vi "CalcFC.vi"(1 "CapUnits":u16(ring) items=["uF", "nF", "pF"], 2 "ResistorUnits":i32(ring) items=["ohm", "Kohm "], 3 "C":ext format="%#_6f", 4 "R":ext format="%#_6f") -> (0 "Fc":ext)   [LabVIEW 2014]
doc: "Calculates the predicted Fc for given Resistor and capacitor values.\nR,C,CapUnits, and ResistorUnits must be wired."
panel:
  out "Tau":ext
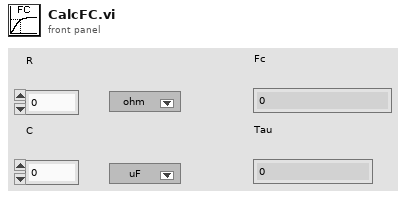
[diagram p1: front panel]
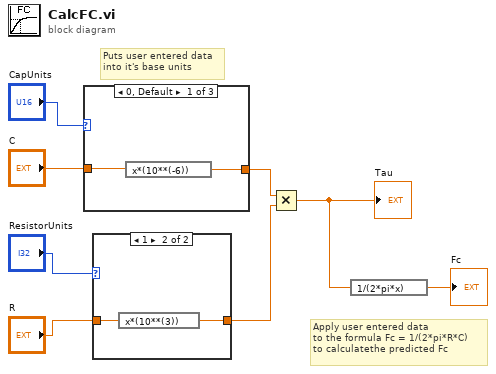
[diagram p0: block diagram]
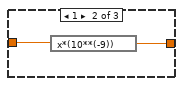
[diagram p3: hidden frame]
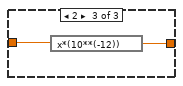
[diagram p4: hidden frame]
diagram:
  # "Apply user entered data\nto the formula Fc = 1/(2*pi*R*C) \nto calculatethe predicted Fc"
  # "Puts user entered data \ninto it's base units"
  n1 = case shown="0, Default" "CapUnits" {
    tunnel: "C" -> [w10 w12 w14]
    tunnel: [w9 w11 w13] -> w3
    frame 0, Default {
      n2 = expression code="x*(10**(-6))"(w10) -> (w9:ext)
    }
    frame 1 {
      n3 = expression code="x*(10**(-9))"(w12) -> (w11:ext)
    }
    frame 2 {
      n4 = expression code="x*(10**(-12))"(w14) -> (w13:ext)
    }
  }
  n5 = case shown="1" "ResistorUnits" {
    tunnel: "R" -> [w15 w17]
    tunnel: [w15 w16] -> w1
    frame 0, Default {
    }
    frame 1 {
      n6 = expression code="x*(10**(3))"(w17) -> (w16:ext)
    }
  }
  n7 = Multiply(x=w3, y=w1) -> (x*y=w8:ext)
  "Tau" <- w8
  n8 = expression code="1/(2*pi*x)"(w8) -> (→"Fc":ext)
